vi "Pre Launch Init.vi"(11 "Topic Actor in":refnum<class "Topic Actor.lvclass">) -> (0 "error out":errorcluster, 3 "Topic Actor out":refnum<class "Topic Actor.lvclass">)   [LabVIEW 2016, in "Stream Mediator.lvlib" / "Topic Actor.lvclass"]
doc: "--\nCopyright © 2017 Composed SystemsI All rights reserved.\n\nAuthor: Jon McBee <jon.mcbee@composed.io>\n\nThis library is provided \"AS IS\" ,WITHOUT WARRANTIES OR\nCONDITIONS OF ANY KIND, either express or implied.\n\nComposed Systems -- composed.io\n\nStream 0.0.1.1\nJon McBee - Composed Systems\nCopyright (c) 2017, Composed Systems"
uses:
  <userlib>/Composed Systems/Stream/Mediator/Classes/Topic Actor/Topic Actor.lvclass
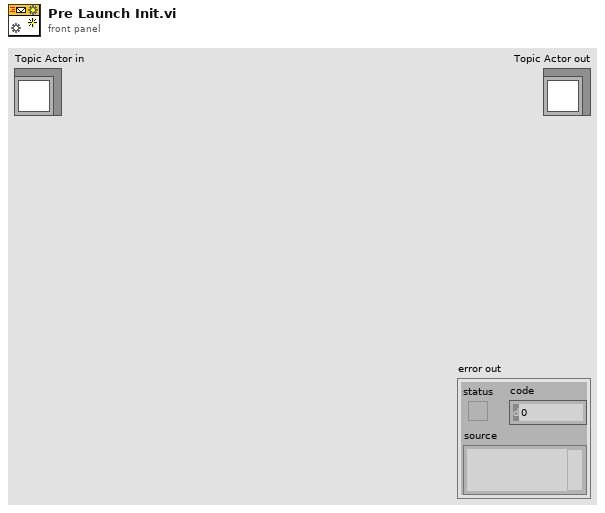
[diagram p1: front panel]
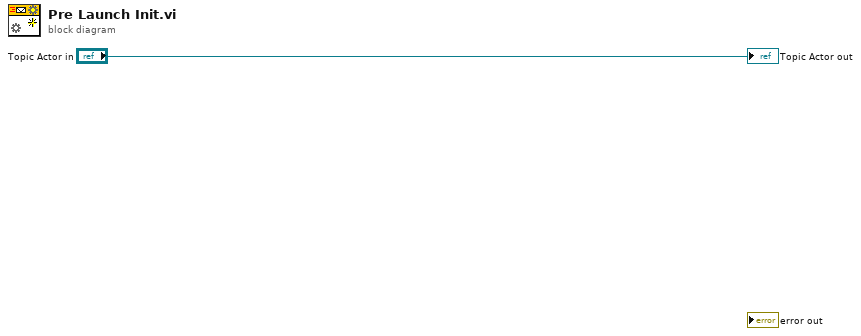
[diagram p0: block diagram]
diagram:
  "Topic Actor out" <- "Topic Actor in"
